vi "SOQPSK Modulator - Channel 0.vi"() -> ()   [LabVIEW 2023]
uses:
  <vilib>/DataMovement_sc/v1/host/Buffer/Buffer v1 Host.lvclass
  <vilib>/rvi/interface/nirviMethod/nirviMethod.xnode
  <vilib>/rvi/interface/nirviCloseFPGA/nirviCloseFPGA.xnode
  <vilib>/rvi/interface/nirviReadWriteControl/nirviReadWriteControl.xnode
  <vilib>/rvi/errors/niLvFpgaMergeErrorWithErrorCode.vi
  <vilib>/rvi/interface/Simulation/niFpgaSimulationCallBeginRW.vi
  <vilib>/rvi/errors/niLvFpgaAdjustHostInterfaceError.vi
  <vilib>/FPGAPlugInAG/Dynamic/niLvFpga_ReadFifo_Dynamic.vi
  Support/Public/FPGA Refnum.ctl
  Support/SOQPSK Host Support.lvlib
  Shared/IRIG106/Host/IRIG106 Filter Generation Host.lvlib
  Shared/IRIG106/Host/IRIG106 SOQPSK Filter Params Type.ctl
  Shared/IRIG106/Host/IRIG106 Signal Type.ctl
  Shared/AWGN/AWGN.lvlib
  <vilib>/addons/Modulation/niDMT.lvlib
  <vilib>/DLsc/v1/Host/Link Engine/DLsc Link Engine v1 Host.lvlib
  <vilib>/FPGAPlugInAG/Dynamic/niLvFpga_Close_Dynamic.vi
  c8235853-d7d8-4eae-95f4-8cb21d7a6b0f.vi
  <vilib>/measure/NI_MAPro.lvlib
  <vilib>/addons/Modulation/Analog/controls/Complex Data Waveform.ctl
  <vilib>/addons/Modulation/niAMT.lvlib
  4451046d-9dee-45a2-a220-eff022c6390e.vi
  <vilib>/Analysis/4window.llb/windowTd.ctl
  <vilib>/Analysis/NI_AALPro.lvlib
  <vilib>/measure/maspectr.llb/FFT Spectrum (Mag-Phase) for 1 Chan (CDB).vi
  <vilib>/DLsc/v1/Host/Link Engine/Commit Links - Single.vi
  <vilib>/DLsc/v1/Host/Protocols/Aurora 64b66b/Extension/Aurora 64b66b Extension.lvlib
  <vilib>/DLsc/v1/Host/Protocols/Aurora 64b66b/Extension/Configure TX - Single.vi
  NiFpgaLv.dll
  <vilib>/Utility/error.llb/Error Cluster From Error Code.vi
  <vilib>/DLsc/v1/Host/Link Engine/Add Hardware - Single.vi
  <vilib>/DLsc/v1/Host/Link Engine/Get Device Registers - IFW.vi
  <vilib>/DLsc/v1/Host/Link Engine/Enable Links - Single.vi
  <vilib>/DLsc/v1/Host/Link Engine/Disable Links - Single.vi
  <vilib>/FPGAPlugInAG/Dynamic/niLvFpga_Download_Dynamic.vi
  <vilib>/FPGAPlugInAG/Dynamic/niLvFpga_Run_Dynamic.vi
  <vilib>/FPGAPlugInAG/Dynamic/niLvFpga_ConfigureFifo_Dynamic.vi
  <vilib>/FPGAPlugInAG/Dynamic/niLvFpga_StartFifo_Dynamic.vi
  <vilib>/FPGAPlugInAG/Dynamic/niLvFpga_WriteFifo_Dynamic.vi
  <vilib>/DLsc/v1/Host/Link Engine/Close References - Single.vi
  Shared/BER/FPGA/PRBS/PRBS Degree Selection.ctl
  Shared/BER/FPGA/PRBS/PRBS.lvlib
  <vilib>/userDefined/High Color/nirio_resource_hc.ctl
panel:
  in  "disable DL":bool
  in  "enable DL":bool
  in  "Trellis Length":i32=4
  in  "Coprocessor Device Name":T1="7903"
  in  "Eb/N0 (dB)":dbl=30.0 min=0.0 max=100.0 step=1.0 format="%.2g"
  out "Trellis Graph":cluster{"t0":dbl, "dt":dbl, "phase":dbl[]}[](graph)
  in  "Autoscale":bool
  in  "FFT Size":i32=1024 caption="FFT size"
  out "FFT Spectrum":cluster{"f0":dbl, "df":dbl, "Y":dbl[]}(graph)={"f0"=-1996093.75, "df"=3906.25, "Y"=[]} caption="SOQPSK Baseband Spectrum"
  out "Bitfile Redownloaded":bool
  in  "Signal Parameters":T3={"Symbol Rate (Hz)"=18000000.0, "Pulse Parameters"={"Payload Length"=500, "Preamble Symbol"=449838109, "PN Order"=0}} {"Pulse Parameters"."PN Order" items=["7", "9", "10", "11", "15", "17", "18", "20", "21", "22", "23", "25"]; "Pulse Parameters"."Preamble Symbol" format="%.0x"; "Symbol Rate (Hz)" format="%#_6p"}
  in  "Coprocessor Bitfile Path":path=path "C:/Users/ADG-RF/Desktop/Modems/soqpsk_modem_dmsc_7903_00_x420_single_channel.lvbitx"
  out "Actual Symbol Rate (Hz)":dbl caption="actual symbol rate" format="%#_6p"
  out "IQ Rate (S/s)":dbl format="%#_6p"
  out "Samples per Symbol":i32
  in  "stop":bool
  out "Status":string
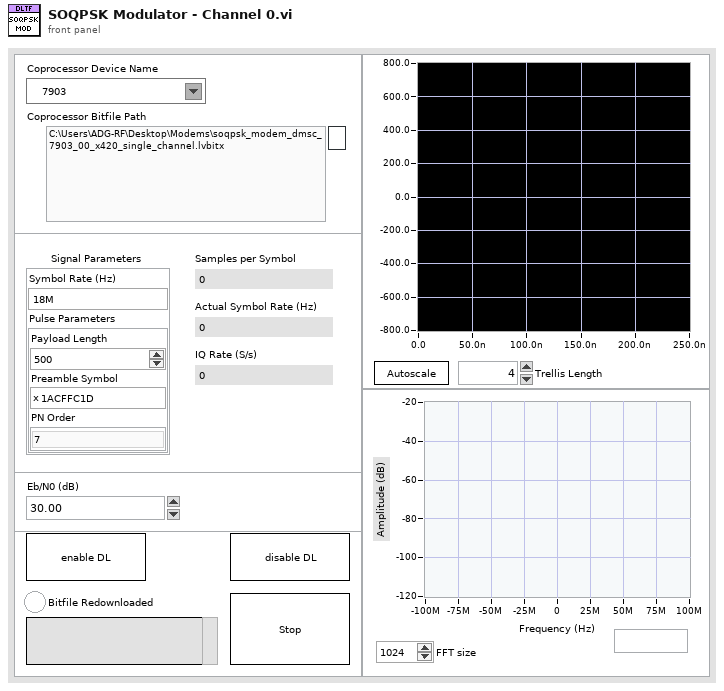
[diagram p1: front panel]
types:
  T1 = typedef "nirio_resource_hc.ctl" = tag
  T2 = typedef "Modems Shared.lvlib/PRBS.lvlib/PRBS Degree Selection.ctl" = u16
  T3 = cluster{"Symbol Rate (Hz)":dbl, "Pulse Parameters":cluster{"Payload Length":u16, "Preamble Symbol":i32, "PN Order":T2}}
  T4 = cluster{"dstepid":u16, "nummdata":fxp<+,5,5>, "pkttype":fxp<+,3,3>, "burst length":u16, "vector length":u16, "vc":fxp<+,6,6>}
  T5 = typedef "SOQPSK Host Support.lvlib/FPGA Refnum.ctl" = refnum<k20>
  T6 = typedef "DLsc Link Engine v1 Host.lvlib/DLsc Session.lvclass/Session Handle.ctl" = refnum<data-value>
  T7 = typedef "DLsc Link Engine v1 Host.lvlib/DLsc Session.lvclass/Device Address Information.ctl" = cluster{"device name":string, "bitfile path":path}
  T8 = typedef "IFW Session v1 Host.lvlib/IFW Session.ctl" = cluster{"refnum":refnum<k20>, "subsystem map":refnum<class "niInstr Subsystem Map v1 Host.lvclass">, "register bus":refnum<class "niInstr FIFO Register Bus v1 Host.lvclass">, "IFW subsystems":T9}
  T9 = typedef "IFW Session v1 Host.lvlib/IFW Subsystems.ctl" = cluster{"IFW address space collection":T10}[]
  T10 = typedef "IFW Session v1 Host.lvlib/IFW Address Space Collection.ctl" = T11[]
  T11 = typedef "IFW Session v1 Host.lvlib/IFW Address Space.ctl" = cluster{"name":string, "IFW address space information":T12, "class path":path}
  T12 = typedef "IFW Session v1 Host.lvlib/IFW Address Space Information.ctl" = cluster{"UID":u16, "instance":u8}
  T13 = cluster{"samples per alpha":u8, "Initial Phase":fxp<+/-,24,1>, "FIR coefficients":fxp<+/-,24,1>[]}
  T14 = typedef "Modems Shared Host.lvlib/IRIG106 Filter Generation Host.lvlib/IRIG106 SOQPSK Filter Params Type.ctl" = enum32{"TG", "MIL", "A", "B", "Custom"}
  T15 = typedef "Modems Shared Host.lvlib/IRIG106 Filter Generation Host.lvlib/IRIG106 Signal Type.ctl" = enum16{"PCM/FM", "SOQPSK-TG", "ARTM CPM"}
  T16 = typedef "Modems Shared Host.lvlib/IRIG106 Filter Generation Host.lvlib/IRIG106 Filter Generation SOQPSK Parameters.ctl" = cluster{"ro":dbl, "B":dbl, "T1":dbl, "T2":dbl}
  T17 = typedef "Modems Shared.lvlib/AWGN.lvlib/Output Type Selection.ctl" = enum16{"I16.1", "I16.2", "I16.3", "I16.4", "I16.5", "AWGN"}
  T18 = typedef "niAMT.lvlib/Complex Data Waveform.ctl" = cluster{"t0":dbl, "dt":dbl, "Y":cdb[]}
  T19 = cluster{"dB On (F)":bool, "unwrap phase (F)":bool, "convert to degree (F)":bool}
  T20 = typedef "NI_AALPro.lvlib/windowTd.ctl" = u32
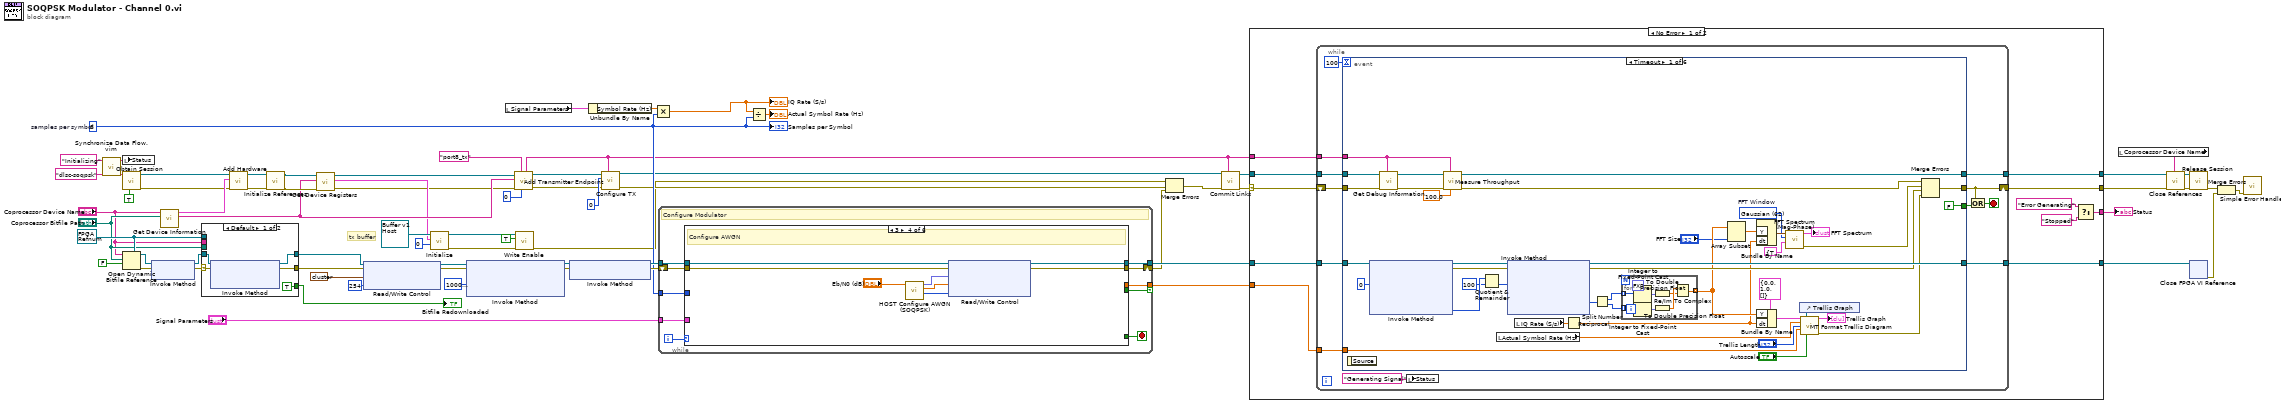
[diagram p0: block diagram]
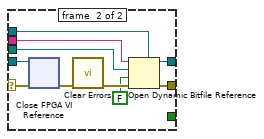
[diagram p2: hidden frame]
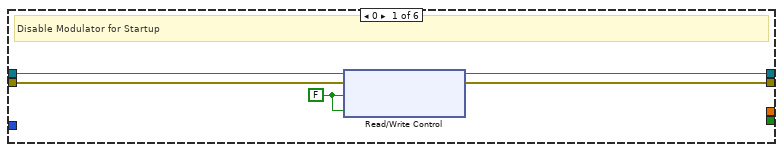
[diagram p3: hidden frame]
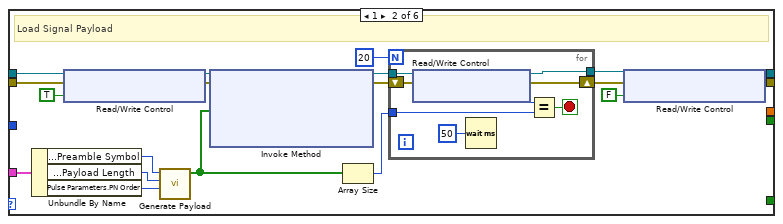
[diagram p4: hidden frame]
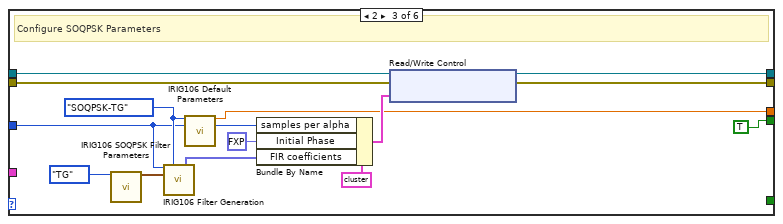
[diagram p5: hidden frame]
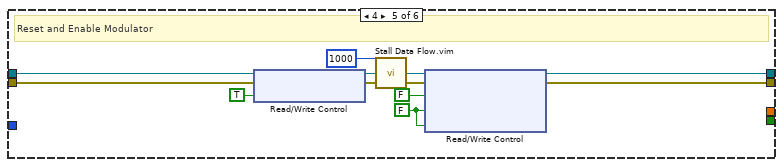
[diagram p6: hidden frame]
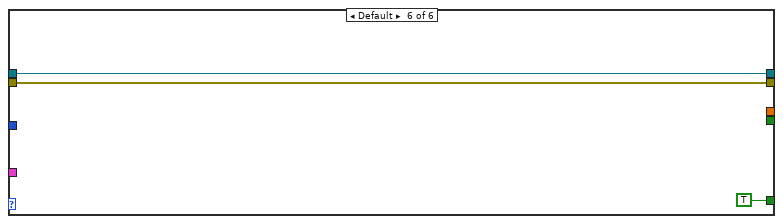
[diagram p7: hidden frame]
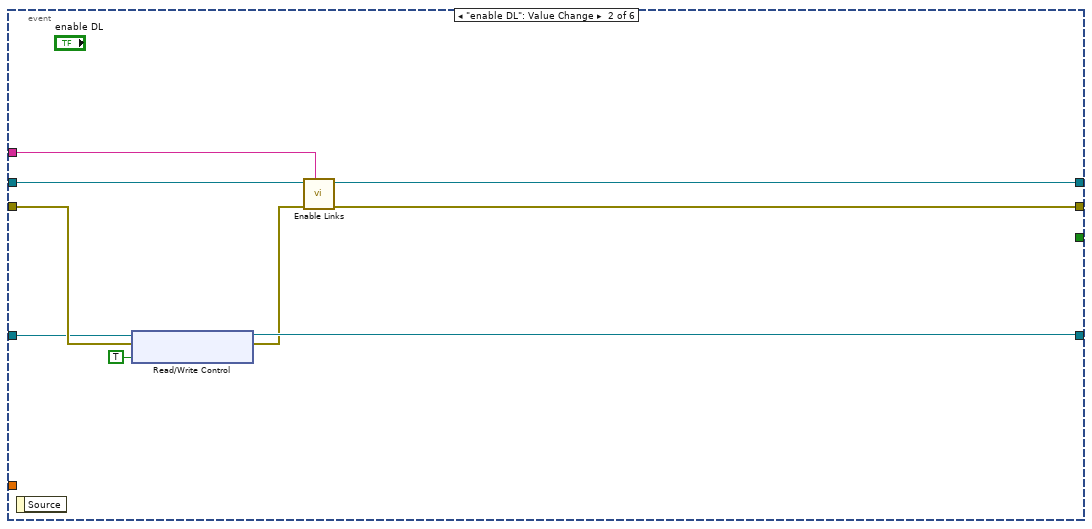
[diagram p8: hidden frame]
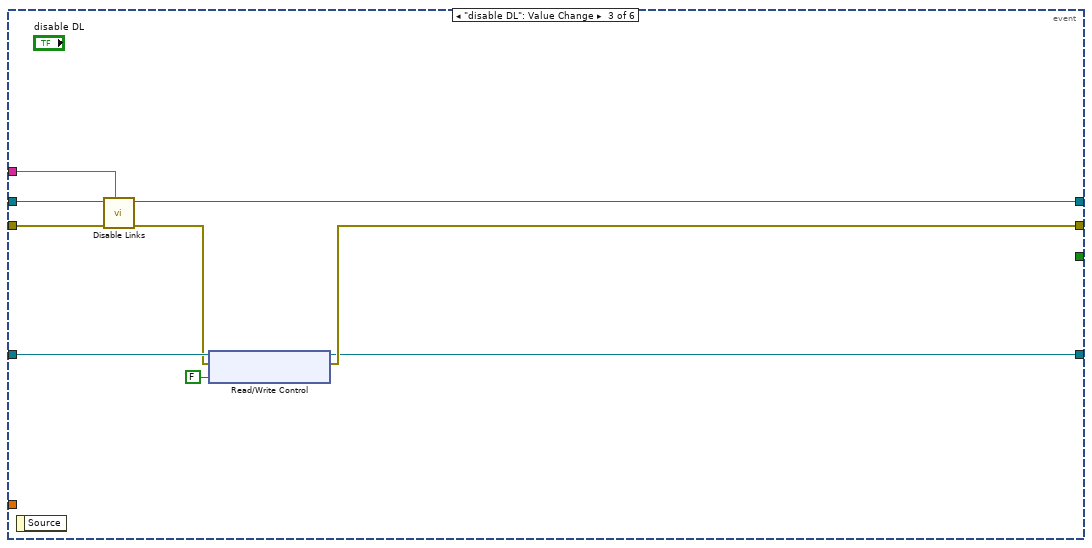
[diagram p9: hidden frame]
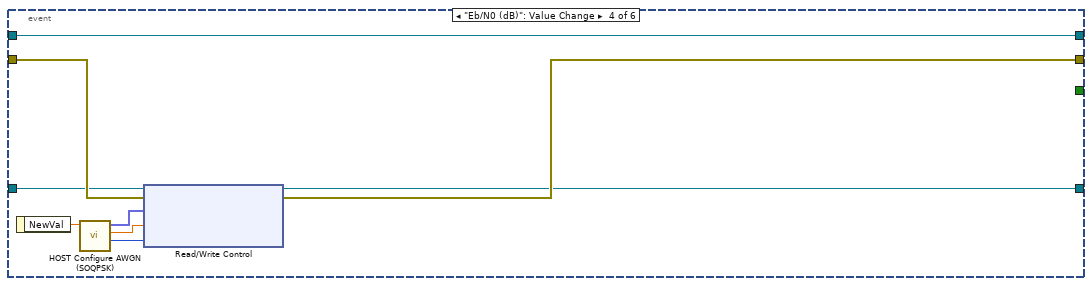
[diagram p10: hidden frame]
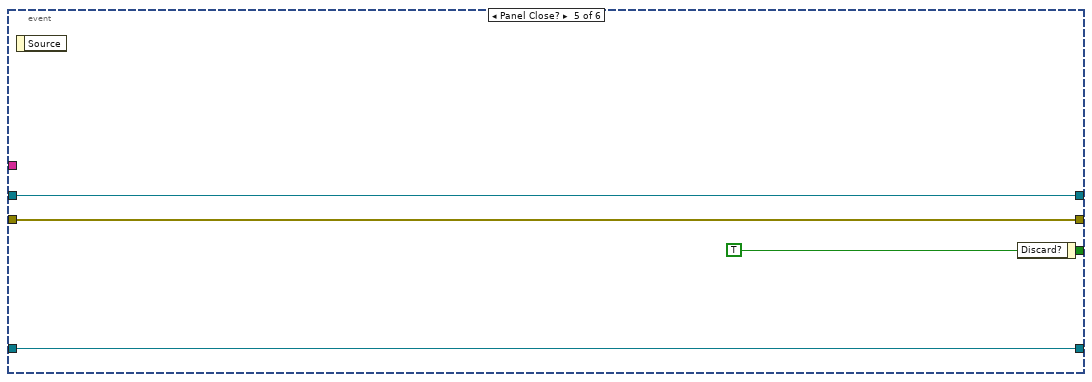
[diagram p11: hidden frame]
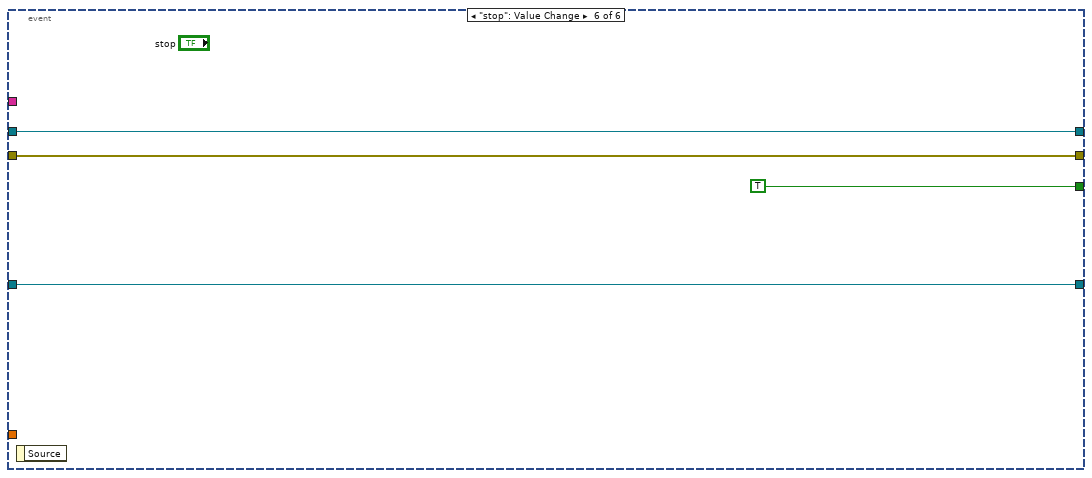
[diagram p12: hidden frame]
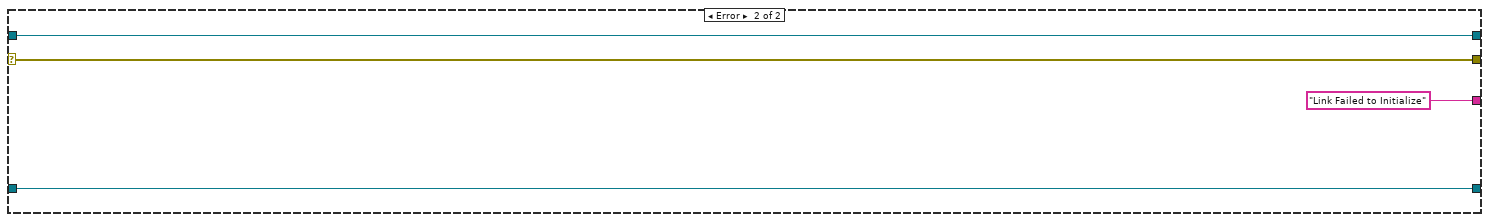
[diagram p13: hidden frame]
diagram:
  w47 = T5 refnum ("datalink soqpsk fpga refnum")
  w58 = 8  # samples per symbol
  # "tx buffer"
  n1 = call "Synchronize Data Flow.vim"("input 4"="dlsc-soqpsk" ("session name"), "input 1"="Initializing") -> ("output 4"=w41:string, "output 1"=w39:string)  [unwired: 2 in, 2 out]
  n2 = local write "Status"(w39) -> ()
  n3 = call <vilib>:"Obtain Session.vi"("use remote engine (f)"=TRUE ("Remote Engine"), "session name (\"\":default)"=w41) -> ("error out"=w23:errorcluster, "session out"=w24:T6)  [unwired: 6 in, 2 out]
  n4 = Open Dynamic Bitfile Reference(0:"Coprocessor Device Name", 1:"Coprocessor Bitfile Path", 2:FALSE ("Run When Loaded"), 4:w47) -> (5:w46:T5, 8:w45:errorcluster)  [unwired: 1 in]
  n5 = xnode "Invoke Method"("FPGA VI Reference In"=w46, "error in"=w45) -> ("FPGA VI Reference Out"=w49:T5, "error out"=w48:errorcluster)
  n6 = call <vilib>:"Get Device Information.vi"("bitfile path"="Coprocessor Bitfile Path", "device name"="Coprocessor Device Name") -> ("device name out"=w12:string, "device address information"=w54:T7)  [unwired: 7 in, 1 out]
  n7 = case shown="Default" w48 {
    selector: w48 -> [w75 w87]
    tunnel: [w77 w80] -> w20
    tunnel: [w76 w83] -> w19
    tunnel: w49 -> [w74 w85]
    tunnel: w47 -> [_ w81]
    tunnel: "Coprocessor Device Name" -> [_ w79]
    tunnel: "Coprocessor Bitfile Path" -> [_ w78]
    tunnel: [TRUE _] -> w38
    frame #0 {
      n8 = xnode "Invoke Method"("FPGA VI Reference In"=w74, "error in"=w75) -> ("FPGA VI Reference Out"=w77:T5, "error out"=w76:errorcluster)  [unwired: 1 in]
    }
    frame #1 {
      n9 = xnode "Close FPGA VI Reference"("FPGA VI Reference In"=w85, "error in"=w87) -> ("error out"=w86:errorcluster)
      n10 = call <vilib>:"Clear Errors.vi"("error in (no error)"=w86) -> ("error out"=w84:errorcluster)  [unwired: 5 in, 1 out]
      n11 = Open Dynamic Bitfile Reference(0:w79, 1:w78, 2:FALSE ("Run When Loaded"), 3:w84, 4:w81) -> (5:w80:T5, 8:w83:errorcluster)
    }
  }
  "Bitfile Redownloaded" <- w38
  n12 = call-poly <vilib>:"Add Hardware.vi"("error in"=w23, "device"=w54, "session in"=w24) -> ("error out"=w15:errorcluster, "session out"=w16:T6)  [unwired: 7 in]
  n13 = call <vilib>:"Initialize References.vi"("error in"=w15, "session in"=w16) -> ("error out"=w13:errorcluster, "session out"=w14:T6)  [unwired: 8 in]
  n14 = call-poly <vilib>:"Get Device Registers.vi"("error in"=w13, "hardware name"=w12, "session in"=w14) -> ("error out"=w5:errorcluster, "ifw session"=w7:T8, "session out"=w6:T6)  [unwired: 6 in]
  n15 = xnode "Read/Write Control"("FPGA VI Reference In"=w20, "error in"=w19, "header parameters.0"=T4 {"dstepid"=777, "nummdata"=0.0, "pkttype"=6.0, "burst length"=506, "vector length"=1012, "vc"=1.0} ("header parameters"), "aurora frame length.0"=u16 254 ("aurora frame length")) -> ("FPGA VI Reference Out"=w22:T5, "error out"=w21:errorcluster)
  n16 = call-dynamic "Initialize.vi"("instance(0)"=u8 0, "session"=w7, "ifw address space collection host in"=refnum<class "Buffer v1 Host.lvclass"> refnum ("Buffer v1 Host.lvclass")) -> ("error out"=w11:errorcluster, "ifw address space collection host out"=w10:refnum<class "Buffer v1 Host.lvclass">)  [unwired: 6 in, 1 out]
  n17 = xnode "Invoke Method"("FPGA VI Reference In"=w22, "error in"=w21, "Requested Depth"=u32 10000000) -> ("FPGA VI Reference Out"=w64:T5, "error out"=w63:errorcluster)  [unwired: 1 out]
  n18 = local read "Signal Parameters"() -> (w43:T3)
  n19 = call <vilib>:"Add Transmitter Endpoint.vi"("transmitter instance (0)"=u8 0, "link name"="port8_tx", "error in"=w5, "transmitter device name"=w12, "session in"=w6) -> ("error out"=w3:errorcluster, "session out"=w4:T6, "link name out"=w25:string)  [unwired: 2 in, 2 out]
  n20 = call <vilib>:"Write Enable.vi"("error in"=w11, "enable (f)"=TRUE, "buffer v1 host in"=w10) -> ("error out"=w2:errorcluster)  [unwired: 7 in, 1 out]
  n21 = xnode "Invoke Method"("FPGA VI Reference In"=w64, "error in"=w63) -> ("FPGA VI Reference Out"=w59:T5, "error out"=w72:errorcluster)
  n22 = Unbundle By Name(w43) -> ("Symbol Rate (Hz)"=w70:dbl)
  n23 = call-poly <vilib>:"Configure TX.vi"("link name (\"\":default)"=w25, "error in"=w3, "frame size"=u16 0 ("tx frame size"), "session in"=w4) -> ("error out"=w26:errorcluster, "session out"=w27:T6)  [unwired: 6 in]
  n24 = Multiply(x=w70, y=w58) -> (x*y=w34:dbl)
  "IQ Rate (S/s)" <- w34
  n25 = while {
    tunnel: [w96] -> w57
    shift-right: [w95] -> w56
    shift-left: w72 -> [w93]
    tunnel: w59 -> [w94]
    tunnel: [w92] -> w55 if=w88
    tunnel: w58 -> [w90]
    tunnel: "Signal Parameters" -> [w89]
    i -> [w97]
    stop <- w91 stop-if-true
    # "Configure Modulator"
    n26 = case shown="3" w97 {
      tunnel: [w100 w111 w135 w150 w157 w166] -> w96
      tunnel: [w99 w110 w134 w149 w156 w165] -> w95
      tunnel: w94 -> [w102 w109 w137 w152 w162 w166]
      tunnel: w93 -> [w101 w108 w136 w151 w161 w165]
      tunnel: [_ _ w132 _ _ _] -> w92
      tunnel: [_ _ _ _ _ TRUE] -> w91
      tunnel: w90 -> [_ _ w131 _ _ _]
      tunnel: w89 -> [_ w104 _ _ _ _]
      tunnel: [_ _ TRUE _ _ _] -> w88
      frame 0 {
        w98 = FALSE ("enable modulator")
        # "Disable Modulator for Startup"
        n27 = xnode "Read/Write Control"("FPGA VI Reference In"=w102, "error in"=w101, "enable modulator.0"=w98, "enable precoder.0"=w98) -> ("FPGA VI Reference Out"=w100:T5, "error out"=w99:errorcluster)
      }
      frame 1 {
        # "Load Signal Payload"
        n28 = Unbundle By Name(w104) -> ("Pulse Parameters.Preamble Symbol"=w105:i32, "Pulse Parameters.Payload Length"=w106:u16, "Pulse Parameters.PN Order"=w107:T2)
        n29 = xnode "Read/Write Control"("FPGA VI Reference In"=w109, "error in"=w108, "update bit generation.0"=TRUE ("update bit generation")) -> ("FPGA VI Reference Out"=w120:T5, "error out"=w119:errorcluster)
        n30 = call "Generate Payload.vi"("PRBS degree"=w107, "payload length"=w106, "preamble symbol"=w105) -> ("bit stream"=w118:bool[])  [unwired: 8 in]
        n31 = xnode "Invoke Method"("FPGA VI Reference In"=w120, "error in"=w119, "Data"=w118) -> ("FPGA VI Reference Out"=w117:T5, "error out"=w116:errorcluster)  [unwired: 1 in, 1 out]
        n32 = Array Size(array=w118) -> (size(s)=w103:i32)
        n33 = for {
          N: 20 -> [_]
          shift-right: [w128] -> w112
          shift-left: w116 -> [w129]
          tunnel: w103 -> [w125]
          tunnel: w117 -> [w127]
          tunnel: [w126] -> w113
          stop <- w122 stop-if-true
          n34 = xnode "Read/Write Control"("FPGA VI Reference In"=w127, "error in"=w129) -> ("FPGA VI Reference Out"=w126:T5, "error out"=w128:errorcluster, "bit stream length.0"=w123:u32)
          n35 = Wait (ms)(milliseconds to wait=u32 50) -> ()  [unwired: 1 out]
          n36 = Equal?(x=w123, y=w125) -> (x = y?=w122:bool)
        }
        n37 = xnode "Read/Write Control"("FPGA VI Reference In"=w113, "error in"=w112, "update bit generation.0"=FALSE ("update bit generation")) -> ("FPGA VI Reference Out"=w111:T5, "error out"=w110:errorcluster)
      }
      frame 2 {
        w140 = IRIG106_Signal_Type."SOQPSK-TG" ("irig106 signal type")
        # "Configure SOQPSK Parameters"
        n38 = call "IRIG106 SOQPSK Filter Parameters.vi"("SOQPSK Filter Params Type"=IRIG106_SOQPSK_Filter_Params_Type."TG") -> ("SOQPSK Filter Params Out"=w139:T16)  [unwired: 14 in]
        n39 = call "IRIG106 Filter Generation.vi"("samples per symbol"=w131, "irig106 signal type"=w140, "soqpsk filter parameters"=w139) -> ("filter fxp"=w142:fxp<+/-,24,1>[])  [unwired: 7 in, 5 out]
        n40 = call "IRIG106 Default Parameters.vi"("IRIG106 Signal Type"=w140, "Samples Per Symbol"=w131) -> ("Modulation Index"=w132:dbl, "samples per alpha"=w143:i32)  [unwired: 7 in, 5 out]
        n41 = Bundle By Name(cluster=T13 {"samples per alpha"=0, "Initial Phase"=0.0, "FIR coefficients"=[0.0, 0.0, 0.0, 0.0, 0.0, 0.0, 0.0, 0.0, 0.0, 0.0, 0.0, 0.0, 0.0, 0.0, 0.0, 0.0, 0.0, 0.0, 0.0, 0.0, 0.0, 0.0, 0.0, 0.0, 0.0, 0.0, 0.0, 0.0, 0.0, 0.0, 0.0, 0.0, 0.0, 0.0, 0.0, 0.0, 0.0, 0.0, 0.0, 0.0, 0.0, 0.0, 0.0, 0.0, 0.0, 0.0, 0.0, 0.0, 0.0, 0.0, 0.0, 0.0, 0.0, 0.0, 0.0, 0.0, 0.0, 0.0, 0.0, 0.0, 0.0, 0.0, 0.0, 0.0, 0.0, 0.0, 0.0, 0.0, 0.0, 0.0, 0.0, 0.0, 0.0, 0.0, 0.0, 0.0, 0.0, 0.0, 0.0, 0.0, 0.0, 0.0, 0.0, 0.0, 0.0, 0.0, 0.0, 0.0, 0.0, 0.0, 0.0, 0.0, 0.0, 0.0, 0.0, 0.0, 0.0, 0.0, 0.0, 0.0, 0.0, 0.0, 0.0, 0.0, 0.0, 0.0, 0.0, 0.0, 0.0, 0.0, 0.0, 0.0, 0.0, 0.0, 0.0, 0.0, 0.0, 0.0, 0.0, 0.0, 0.0, 0.0, 0.0, 0.0, 0.0, 0.0, 0.0, 0.0]} ("SOQPSK Parameters"), "samples per alpha"=w143, "Initial Phase"=fxp<+/-,24,1> 0.0, "FIR coefficients"=w142) -> (w133:T13)
        n42 = xnode "Read/Write Control"("FPGA VI Reference In"=w137, "error in"=w136, "soqpsk parameters.0"=w133) -> ("FPGA VI Reference Out"=w135:T5, "error out"=w134:errorcluster)
      }
      frame 3 {
        # "Configure AWGN"
        n43 = call "HOST Configure AWGN (SOQPSK).vi"("E0/Nb"="Eb/N0 (dB)") -> ("output type selection"=w146:T17, "noise std deviation\n(unity signal power)"=w147:dbl, "AWGN seeds"=w148:fxp<+,25,25>[])  [unwired: 8 in]
        n44 = xnode "Read/Write Control"("FPGA VI Reference In"=w152, "error in"=w151, "AWGN seeds.0"=w148, "scaling factor.0"=w147, "output type selection.0"=w146) -> ("FPGA VI Reference Out"=w150:T5, "error out"=w149:errorcluster)
      }
      frame 4 {
        w153 = FALSE ("enable precoder")
        # "Reset and Enable Modulator"
        n45 = xnode "Read/Write Control"("FPGA VI Reference In"=w162, "error in"=w161, "reset modulator.0"=TRUE ("reset modulator")) -> ("FPGA VI Reference Out"=w159:T5, "error out"=w158:errorcluster)
        n46 = call "Stall Data Flow.vim"("value in"=w159, "milliseconds to wait"=u32 1000) -> ("value out"=w155:T5)  [unwired: 1 out]
        n47 = xnode "Read/Write Control"("FPGA VI Reference In"=w155, "error in"=w158, "reset modulator.0"=FALSE ("reset modulator"), "enable modulator.0"=w153, "enable precoder.0"=w153) -> ("FPGA VI Reference Out"=w157:T5, "error out"=w156:errorcluster)
      }
      frame Default {
      }
    }
  }
  n48 = Divide(x=w34, y=w58) -> (x/y=→"Actual Symbol Rate (Hz)":dbl)
  n49 = Merge Errors(w2, w26, w56) -> (w29:errorcluster)
  n50 = call-poly <vilib>:"Commit Links.vi"("link name (\"\":all)"=w25, "error in"=w29, "session in"=w27) -> ("error out"=w60:errorcluster, "session out"=w61:T6)  [unwired: 7 in]
  n51 = case shown="No Error" w60 {
    selector: w60 -> [w169 w276]
    tunnel: w61 -> [w170 w277]
    tunnel: [w168 w277] -> w33
    tunnel: w57 -> [w177 w275]
    tunnel: [w167 w276] -> w32
    tunnel: [w176 w275] -> w68
    tunnel: w55 -> [w175 _]
    tunnel: [w172 "Link Failed to Initialize" ("t")] -> w69
    tunnel: w25 -> [w171 _]
    frame No Error {
      n52 = while {
        shift-right: [w184] -> w167
        shift-left: w169 -> [w189]
        tunnel: w170 -> [w183]
        tunnel: [w182] -> w168
        tunnel: w177 -> [w181]
        tunnel: [w180] -> w176
        tunnel: w175 -> [w179]
        tunnel: w171 -> [w178]
        stop <- w185 stop-if-true
        n53 = event shown="[0] Timeout" {
          selector: _ -> [_ _ _ _ _ _]
          dyn-events: _ -> [_ _ _ _ _ _]
          timeout: 100 ("milliseconds to wait") -> [_ _ _ _ _ _]
          tunnel: w189 -> [w198 w243 w255 w265 w269 w272]
          tunnel: [FALSE ("done?") _ _ _ w266 TRUE ("done?")] -> w188
          tunnel: [w230 w239 w249 w264 w269 w272] -> w184
          tunnel: w183 -> [w199 w247 w256 w261 w267 w271]
          tunnel: [w196 w246 w250 w261 w267 w271] -> w182
          tunnel: w181 -> [w225 w242 w252 w263 w268 w270]
          tunnel: [w227 w241 w248 w262 w268 w270] -> w180
          tunnel: w179 -> [w218 _ _ _ _ _]
          tunnel: w178 -> [w197 w245 w254 _ _ _]
          event Timeout {
            w215 = T20 62 items=["Rectangle"=0, "Hanning"=1, "Hamming"=2, "Blackman-Harris"=3, "Exact Blackman"=4, "Blackman"=5, "Flat Top"=6, "4 Term B-Harris "=7, "7 Term B-Harris"=8, "Low Sidelobe"=9, "Blackman Nuttall"=11, "Triangle"=30, "Bartlett-Hanning"=31, "Bohman"=32, "Parzen"=33, "Welch"=34, "Kaiser"=60, "Dolph-Chebyshev"=61, "Gaussian"=62]  # FFT Window
            n54 = event-data() -> ()  [unwired: 1 in, 1 out]
            n55 = xnode "Invoke Method"("FPGA VI Reference In"=w225, "Number of Elements"=u32 0) -> ("FPGA VI Reference Out"=w229:T5, "error out"=w228:errorcluster, "Elements Remaining"=w192:u32)  [unwired: 2 in, 1 out]
            n56 = call <vilib>:"Get Debug Information.vi"("link name"=w197, "error in"=w198, "session in"=w199) -> ("error out"=w201:errorcluster, "session out"=w200:T6)  [unwired: 5 in, 2 out]
            n57 = call <vilib>:"Measure Throughput.vi"("measurement interval (500ms)"=100.0 ("thruput meas time (ms)"), "link name"=w197, "error in"=w201, "session in"=w200) -> ("error out"=w195:errorcluster, "session out"=w196:T6)  [unwired: 4 in, 2 out]
            n58 = Quotient & Remainder(x=w192, y=u32 100) -> (floor(x/y)=w190:u32)  [unwired: 1 out]
            n59 = local read "Actual Symbol Rate (Hz)"() -> (w205:dbl)
            n60 = xnode "Invoke Method"("FPGA VI Reference In"=w229, "error in"=w228, "Number of Elements"=w190) -> ("FPGA VI Reference Out"=w227:T5, "error out"=w226:errorcluster, "Data"=w193:u32[])  [unwired: 1 in, 1 out]
            n61 = local read "IQ Rate (S/s)"() -> (w207:dbl)
            n62 = Reciprocal(x=w207) -> (1/x=w206:dbl)
            n63 = Split Number(x=w193) -> (hi(x)=w224:u16[], lo(x)=w223:u16[])
            n64 = for {
              tunnel: w224 -> [w238] mode=indexing
              tunnel: w223 -> [w237] mode=indexing
              tunnel: [w234] -> w210 mode=indexing
              w231 = fxp<+/-,16,1> 0.0 ("fixed-point type")
              n65 = Integer to Fixed-Point Cast(fixed-point type=w231, integer=w238) -> (fixed-point=w236:fxp<+/-,16,1>)
              n66 = Integer to Fixed-Point Cast(fixed-point type=w231, integer=w237) -> (fixed-point=w235:fxp<+/-,16,1>)
              n67 = To Double Precision Float(number=w236) -> (double precision float=w232:dbl)
              n68 = To Double Precision Float(number=w235) -> (double precision float=w233:dbl)
              n69 = Re/Im To Complex(1:w232, 2:w233) -> (0:w234:cdb)
            }
            n70 = Array Subset(array=w210, length="FFT Size") -> (w211:cdb[])  [unwired: 1 in]
            n71 = Bundle By Name("Y"=w211, "dt"=w206) -> (w216:waveform(cdb))  [unwired: 1 in]
            n72 = Bundle By Name(cluster=T18 {"t0"=0.0, "dt"=1.0, "Y"=[]} ("waveform"), "Y"=w210, "dt"=w206) -> (w212:T18)
            n73 = call-poly <vilib>:"FFT Spectrum (Mag-Phase).vi"("view"=T19 {"dB On (F)"=TRUE, "unwrap phase (F)"=FALSE, "convert to degree (F)"=FALSE}, "window"=w215, "time signal"=w216) -> ("error out"=w208:errorcluster, "magnitude"=→"FFT Spectrum":cluster{"f0":dbl, "df":dbl, "magnitude":dbl[]})  [unwired: 4 in, 3 out]
            n74 = control-ref of="Trellis Graph"() -> (w221:refnum<vi>)
            n75 = call <vilib>:"MT Format Trellis Diagram.vi"("waveform"=w212, "trellis reference"=w221, "symbol rate (Hz)"=w205, "trellis length"="Trellis Length", "modulation index"=w218, "autoscale"="Autoscale") -> ("trellis diagram"=→"Trellis Graph":cluster{"t0":dbl, "dt":dbl, "phase":dbl[]}[], "error out"=w219:errorcluster)  [unwired: 1 in, 7 out]
            n76 = Merge Errors(w195, w208, w226, w219) -> (w230:errorcluster)
          }
          event "enable DL": Value Change {
            n77 = event-data() -> ()  [unwired: 1 in, 1 out]
            n78 = xnode "Read/Write Control"("FPGA VI Reference In"=w242, "error in"=w243, "enable modulator.0"=TRUE ("enable modulator")) -> ("FPGA VI Reference Out"=w241:T5, "error out"=w240:errorcluster)
            n79 = call-poly <vilib>:"Enable Links.vi"("link name (\"\":all)"=w245, "error in"=w240, "session in"=w247) -> ("error out"=w239:errorcluster, "session out"=w246:T6)  [unwired: 7 in]
          }
          event "disable DL": Value Change {
            n80 = event-data() -> ()  [unwired: 1 in, 1 out]
            n81 = call-poly <vilib>:"Disable Links.vi"("link name (\"\":all)"=w254, "error in"=w255, "session in"=w256) -> ("error out"=w251:errorcluster, "session out"=w250:T6)  [unwired: 7 in]
            n82 = xnode "Read/Write Control"("FPGA VI Reference In"=w252, "error in"=w251, "enable modulator.0"=FALSE ("enable modulator")) -> ("FPGA VI Reference Out"=w248:T5, "error out"=w249:errorcluster)
          }
          event "Eb/N0 (dB)": Value Change {
            n83 = event-data() -> ("NewVal"=w260:dbl)  [unwired: 1 in]
            n84 = call "HOST Configure AWGN (SOQPSK).vi"("E0/Nb"=w260) -> ("output type selection"=w258:T17, "noise std deviation\n(unity signal power)"=w259:dbl, "AWGN seeds"=w257:fxp<+,25,25>[])  [unwired: 8 in]
            n85 = xnode "Read/Write Control"("FPGA VI Reference In"=w263, "error in"=w265, "AWGN seeds.0"=w257, "scaling factor.0"=w259, "output type selection.0"=w258) -> ("FPGA VI Reference Out"=w262:T5, "error out"=w264:errorcluster)
          }
          event Panel Close? {
            w266 = TRUE
            n86 = event-data() -> ()  [unwired: 1 in, 1 out]
            n87 = event-data("Discard?"=w266) -> ()  [unwired: 1 in, 1 out]
          }
          event "stop": Value Change {
            n88 = event-data() -> ()  [unwired: 1 in, 1 out]
          }
        }
        n89 = local write "Status"("Generating Signal" ("Status")) -> ()
        n90 = Or(x=w184, y=w188) -> (x .or. y?=w185:bool)
      }
      n91 = Select(t="Error Generating", s=w167, f="Stopped") -> (s? t:f=w172:string)
    }
    frame Error {
    }
  }
  "Status" <- w69
  n92 = local read "Coprocessor Device Name"() -> (w35:T1)
  n93 = call-poly <vilib>:"Close References.vi"("device name"=w35, "error in"=w32, "session in"=w33) -> ("error out"=w52:errorcluster, "session out"=w53:T6)  [unwired: 7 in]
  n94 = call <vilib>:"Release Session.vi"("error in"=w52, "session in"=w53) -> ("error out"=w51:errorcluster)  [unwired: 8 in, 1 out]
  n95 = xnode "Close FPGA VI Reference"("FPGA VI Reference In"=w68) -> ("error out"=w66:errorcluster)  [unwired: 1 in]
  n96 = Merge Errors(w51, w66) -> (w67:errorcluster)
  n97 = call <vilib>:"Simple Error Handler.vi"("error in (no error)"=w67) -> ()  [unwired: 4 in, 5 out]
  "Samples per Symbol" <- w58
